vi "receive messages.vi"(8 "error in (no error)":errorcluster, 11 "Header content in":refnum<class "Header content.lvclass">) -> (0 "error out":errorcluster, 3 "Header content out":refnum<class "Header content.lvclass">)   [LabVIEW 2018, in "Header content.lvclass"]
uses:
  Header content.lvclass
  Header content.lvclass/Header content.ctl
  Server/Server.lvclass
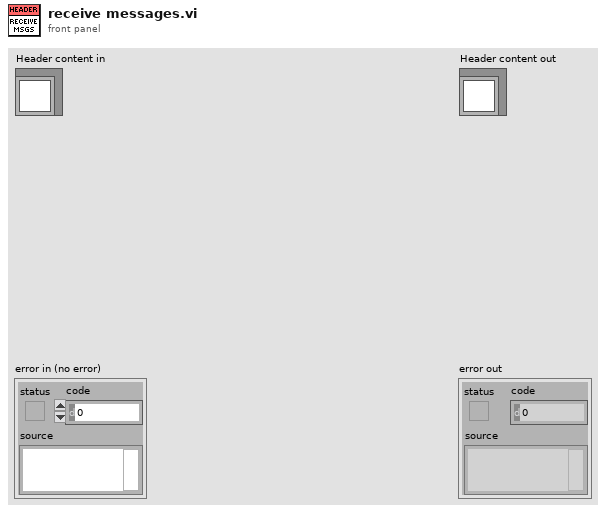
[diagram p1: front panel]
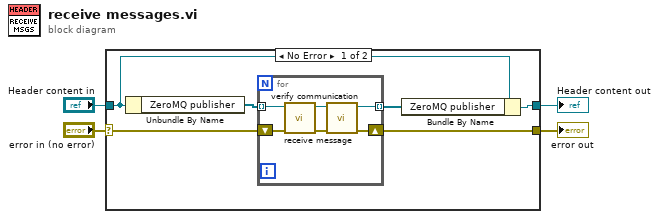
[diagram p0: block diagram]
diagram:
  n1 = case shown="No Error" "error in (no error)" {
    selector: "error in (no error)" -> [w10 w18]
    tunnel: [w9 w18] -> w3
    tunnel: [w7 w17] -> w1
    tunnel: "Header content in" -> [w8 w17]
    frame No Error {
      n2 = Unbundle By Name(w8) -> ("ZeroMQ publisher"=w5:refnum<class "Server.lvclass">[])
      n3 = for {
        shift-right: [w12] -> w9
        shift-left: w10 -> [w15]
        tunnel: [w11] -> w6 mode=indexing
        tunnel: w5 -> [w16] mode=indexing
        n4 = call "receive message.vi"("error in (no error)"=w15, "Server in"=w16) -> ("error out"=w13:errorcluster, "Server out"=w14:refnum<class "Server.lvclass">)  [unwired: 8 in]
        n5 = call "verify communication.vi"("error in (no error)"=w13, "Server in"=w14) -> ("error out"=w12:errorcluster, "Server out"=w11:refnum<class "Server.lvclass">)  [unwired: 8 in]
      }
      n6 = Bundle By Name(cluster=w8, "ZeroMQ publisher"=w6) -> (w7:refnum<class "Header content.lvclass">)
    }
    frame Error {
    }
  }
  "error out" <- w3
  "Header content out" <- w1
